vi "Initialize.vi"(8 "error in (no error)":errorcluster, 9 "Reset (True)":bool=TRUE, 10 "ID Query (True)":bool=TRUE, 11 "VISA resource name":refnum<visa-resource-name>) -> (0 "error out":errorcluster, 3 "VISA resource name out":refnum<visa-resource-name>)   [LabVIEW 2019, in "Pendulum CNT90.lvlib"]
doc: "Establishes communication with the instrument and optionally performs an instrument identification query and/or an instrument reset. It also places the instrument in a default state needed for other instrument driver operations. Therefore, call this VI before calling other instrument driver VIs for this instrument. Generally, you need to call the <B>Initialize VI</B> only once at the beginning of an application."
uses:
  Pendulum CNT90.lvlib
panel:
  # "(c) 2007 National Instruments.  ALL RIGHTS RESERVED."
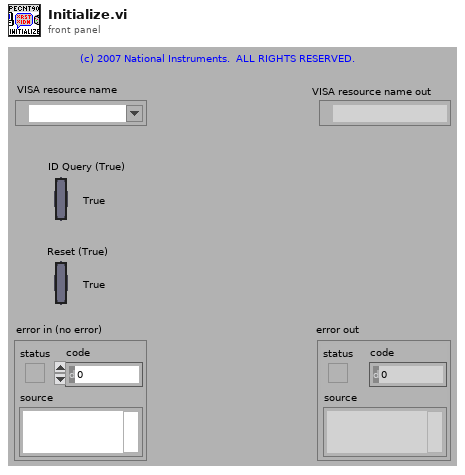
[diagram p1: front panel]
types:
  T1 = cluster{"Status":bool, "Code":i32, "Source (VI Name)":string}
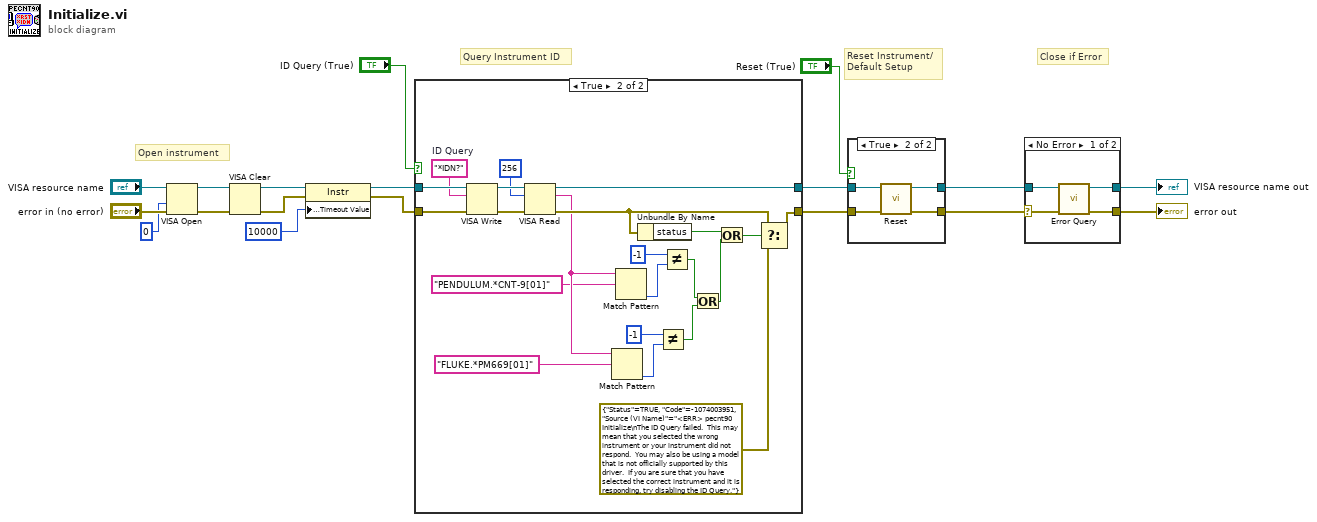
[diagram p0: block diagram]
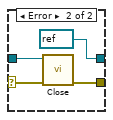
[diagram p2: hidden frame]
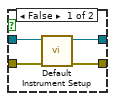
[diagram p3: hidden frame]
diagram:
  # "Close if Error"
  # "Query Instrument ID"
  # "Reset Instrument/\nDefault Setup"
  # "Open instrument"
  n1 = VISA Open(access mode=u32 0, error in (no error)="error in (no error)", VISA resource name="VISA resource name") -> (VISA resource name=w8:refnum<visa-resource-name>, error out=w7:errorcluster)  [unwired: 2 in]
  n2 = VISA Clear(VISA resource name=w8, error in (no error)=w7) -> (VISA resource name out=w6:refnum<visa-resource-name>, error out=w5:errorcluster)
  n3 = property class="Instr"(reference=w6, error in=w5, "General Settings:Timeout Value"=u32 10000) -> (reference out=w11:refnum<visa-resource-name>, error out=w10:errorcluster)
  n4 = case shown="True" "ID Query (True)" {
    tunnel: [w19 w42] -> w17
    tunnel: [w20 w39] -> w18
    tunnel: w11 -> [w20 w40]
    tunnel: w10 -> [w19 w41]
    frame False {
    }
    frame True {
      w30 = "*IDN?"  # ID Query
      n5 = VISA Write(VISA resource name=w40, write buffer=w30, error in (no error)=w41) -> (VISA resource name out=w38:refnum<visa-resource-name>, error out=w36:errorcluster)  [unwired: 1 out]
      n6 = VISA Read(VISA resource name=w38, byte count=u32 256, error in (no error)=w36) -> (VISA resource name out=w39:refnum<visa-resource-name>, read buffer=w23:string, error out=w37:errorcluster)  [unwired: 1 out]
      n7 = Match Pattern(string=w23, regular expression="FLUKE.*PM669[01]") -> (offset past match=w27:i32)  [unwired: 1 in, 3 out]
      n8 = Match Pattern(string=w23, regular expression="PENDULUM.*CNT-9[01]") -> (offset past match=w32:i32)  [unwired: 1 in, 3 out]
      n9 = Unbundle By Name(w37) -> ("status"=w34:bool)
      n10 = Not Equal?(x=-1, y=w27) -> (x != y?=w25:bool)
      n11 = Not Equal?(x=-1, y=w32) -> (x != y?=w26:bool)
      n12 = Or(x=w26, y=w25) -> (x .or. y?=w24:bool)
      n13 = Or(x=w34, y=w24) -> (x .or. y?=w35:bool)
      n14 = Select(t=w37, s=w35, f=T1 {"Status"=TRUE, "Code"=-1074003951, "Source (VI Name)"="<ERR> pecnt90 Initialize\nThe ID Query failed.  This may mean that you selected the wrong instrument or your instrument did not respond.  You may also be using a model that is not officially supported by this driver.  If you are sure that you have selected the correct instrument and it is responding, try disabling the ID Query."}) -> (s? t:f=w42:T1)
    }
  }
  n15 = case shown="True" "Reset (True)" {
    tunnel: w17 -> [w45 w47]
    tunnel: [w44 w50] -> w1
    tunnel: w18 -> [w46 w48]
    tunnel: [w43 w49] -> w2
    frame False {
      n16 = call "Default Instrument Setup.vi"("error in (no error)"=w45, "VISA resource name"=w46) -> ("error out"=w44:errorcluster, "VISA resource name out"=w43:refnum<visa-resource-name>)  [unwired: 8 in]
    }
    frame True {
      n17 = call "Reset.vi"("error in (no error)"=w47, "VISA resource name"=w48) -> ("error out"=w50:errorcluster, "VISA resource name out"=w49:refnum<visa-resource-name>)  [unwired: 8 in]
    }
  }
  n18 = case shown="No Error" w1 {
    selector: w1 -> [w52 w56]
    tunnel: w2 -> [w51 w57]
    tunnel: [w54 refnum<visa-resource-name> refnum ("VISA resource name out")] -> w4
    tunnel: [w53 w58] -> w3
    frame No Error {
      n19 = call "Error Query.vi"("error in (no error)"=w52, "VISA resource name"=w51) -> ("error out"=w53:errorcluster, "VISA resource name out"=w54:refnum<visa-resource-name>)  [unwired: 6 in, 2 out]
    }
    frame Error {
      n20 = call "Close.vi"("error in (no error)"=w56, "VISA resource name"=w57) -> ("error out"=w58:errorcluster)  [unwired: 9 in]
    }
  }
  "VISA resource name out" <- w4
  "error out" <- w3
